vi "PWMOutputEnControl.vi"(8 "ErrorIn(no error)":errorcluster, 10 "OutEN?(F)":bool, 11 "FPGA VI引用输入":refnum<k20>) -> (0 "ErrorOut":errorcluster, 3 "FPGA VI引用输出":refnum<k20>)   [LabVIEW 2015]
uses:
  <vilib>/Utility/error.llb/Error Cluster From Error Code.vi
  <vilib>/rvi/errors/niLvFpgaAdjustHostInterfaceError.vi
  <vilib>/rvi/interface/nirviReadWriteControl/nirviReadWriteControl.xnode
  NiFpgaLv.dll
  <vilib>/rvi/interface/Simulation/niFpgaSimulationCallBeginRW.vi
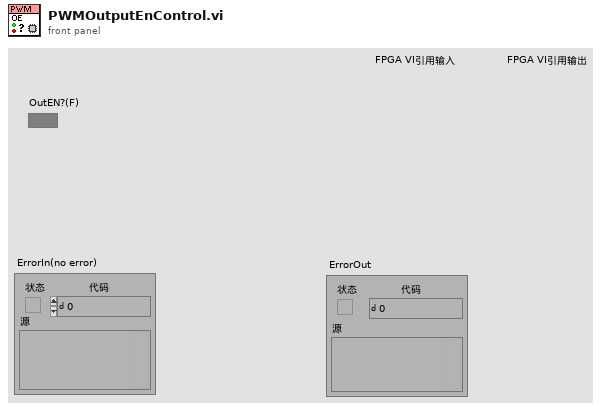
[diagram p1: front panel]
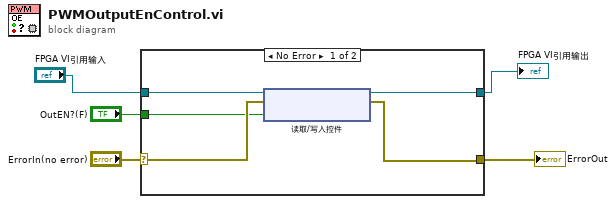
[diagram p0: block diagram]
diagram:
  n1 = case shown="No Error" "ErrorIn(no error)" {
    selector: "ErrorIn(no error)" -> [w9 w11]
    tunnel: "FPGA VI引用输入" -> [w10 w12]
    tunnel: [w8 w12] -> w1
    tunnel: [w7 w11] -> w4
    tunnel: "OutEN?(F)" -> [w6 _]
    frame No Error {
      n2 = xnode "读取/写入控件"("FPGA VI Reference In"=w10, "error in"=w9, "PWMOutputEN"=w6) -> ("FPGA VI Reference Out"=w8:refnum<k20>, "error out"=w7:errorcluster)
    }
    frame Error {
    }
  }
  "ErrorOut" <- w4
  "FPGA VI引用输出" <- w1
